vi "Program_initial.vi"(8 "error in (no error)":errorcluster, 11 "Reference":T1) -> (0 "error out":errorcluster, 3 "dup Reference":T1)   [LabVIEW 2020]
uses:
  Button_Reference.ctl
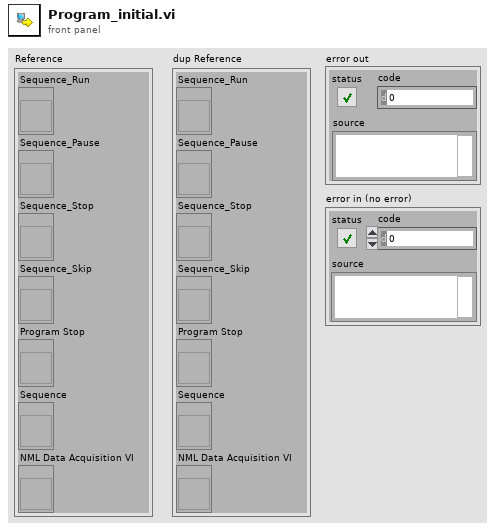
[diagram p1: front panel]
types:
  T1 = typedef "Button_Reference.ctl" = cluster{"Sequence_Run":refnum<vi>, "Sequence_Pause":refnum<vi>, "Sequence_Stop":refnum<vi>, "Sequence_Skip":refnum<vi>, "Program Stop":refnum<vi>, "Sequence":refnum<vi>, "NML Data Acquisition VI":refnum<vi>}
  T2 = enum8{"Enabled", "Disabled", "Disabled and Grayed Out"}
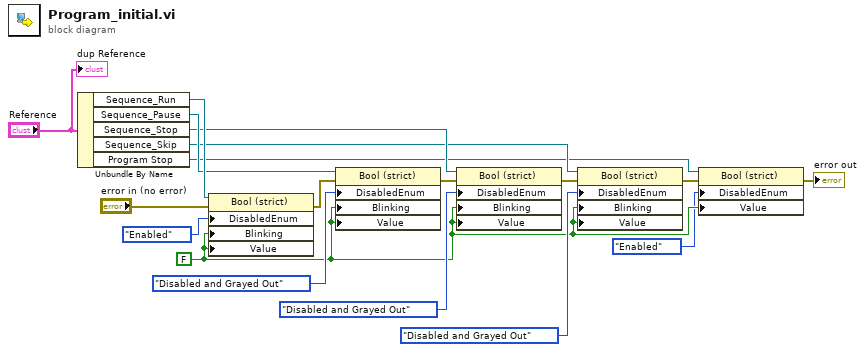
[diagram p0: block diagram]
diagram:
  w8 = FALSE ("Blinking")
  n1 = Unbundle By Name("Reference") -> ("Sequence_Run"=w5:refnum<vi>, "Sequence_Pause"=w4:refnum<vi>, "Sequence_Stop"=w3:refnum<vi>, "Sequence_Skip"=w2:refnum<vi>, "Program Stop"=w1:refnum<vi>)
  n2 = property on="Property Node" class="Bool (strict)"(reference=w5, error in="error in (no error)", "DisabledEnum"=T2."Enabled" ("Disabled"), "Blinking"=w8, "Value"=w8) -> (error out=w11:errorcluster)  [unwired: 1 out]
  n3 = property on="Property Node" class="Bool (strict)"(reference=w4, error in=w11, "DisabledEnum"=T2."Disabled and Grayed Out" ("Disabled"), "Blinking"=w8, "Value"=w8) -> (error out=w12:errorcluster)  [unwired: 1 out]
  n4 = property on="Property Node" class="Bool (strict)"(reference=w3, error in=w12, "DisabledEnum"=T2."Disabled and Grayed Out" ("Disabled"), "Blinking"=w8, "Value"=w8) -> (error out=w16:errorcluster)  [unwired: 1 out]
  n5 = property on="Property Node" class="Bool (strict)"(reference=w2, error in=w16, "DisabledEnum"=T2."Disabled and Grayed Out" ("Disabled"), "Blinking"=w8, "Value"=w8) -> (error out=w18:errorcluster)  [unwired: 1 out]
  n6 = property on="Property Node" class="Bool (strict)"(reference=w1, error in=w18, "DisabledEnum"=T2."Enabled" ("Disabled"), "Value"=w8) -> (error out=→"error out":errorcluster)  [unwired: 1 out]
  "dup Reference" <- "Reference"
